vi "Psychrmoetric Chart by WB.vi"() -> (0 "Psych Chart by WB":dbl[][](array[numeric]))   [LabVIEW 2020]
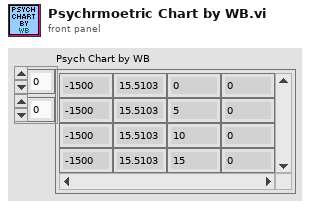
[diagram p1: front panel]
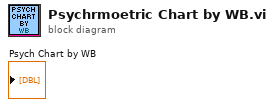
[diagram p0: block diagram]
diagram:
